vi "RectangleToCenter.vi"(11 "rectangle":cluster{i32, i32, i32, i32}={253, 74, 453, 274}) -> (1 "hight":i32, 2 "width":i32, 3 "center":cluster{i32, i32})   [LabVIEW 2011]
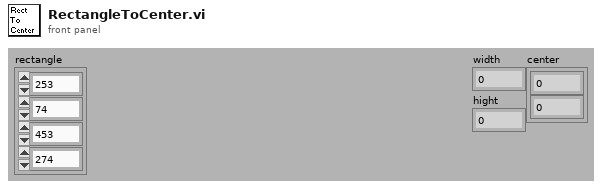
[diagram p1: front panel]
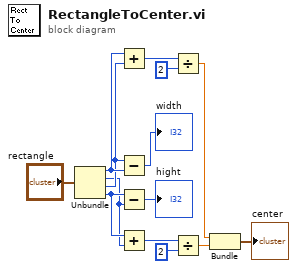
[diagram p0: block diagram]
diagram:
  n1 = Unbundle("rectangle") -> (w11:i32, w2:i32, w10:i32, w3:i32)
  n2 = Add(x=w11, y=w10) -> (x+y=w9:i32)
  n3 = Subtract(x=w10, y=w11) -> (x-y=→"width":i32)
  n4 = Subtract(x=w3, y=w2) -> (x-y=→"hight":i32)
  n5 = Add(x=w3, y=w2) -> (x+y=w4:i32)
  n6 = Divide(x=w9, y=2) -> (x/y=w7:dbl)
  n7 = Divide(x=w4, y=2) -> (x/y=w1:dbl)
  n8 = Bundle(w7, w1) -> (→"center":cluster{dbl, dbl})  [unwired: 1 out]
